vi "ifr2025 RF State.vi"(8 "error in (no error)":errorcluster {"code" format="%.0x"}, 9 "RF State (On)":bool=TRUE, 11 "instrument handle":refnum<visa-resource-name>) -> (0 "error out":errorcluster {"code" format="%.0x"}, 3 "instrument handle out":refnum<visa-resource-name>)   [LabVIEW 2009]
doc: "Controls the instrument RF output."
uses:
  Ifr2025_32.dll
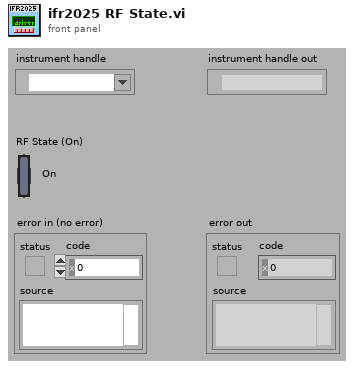
[diagram p1: front panel]
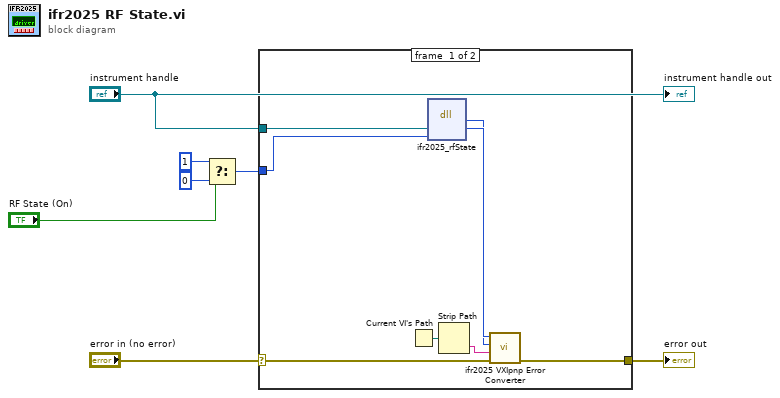
[diagram p0: block diagram]
diagram:
  n1 = Select(t=i16 1, s="RF State (On)", f=i16 0) -> (s? t:f=w1:i16)
  n2 = case shown="No Error" "error in (no error)" {
    selector: "error in (no error)" -> [w10 w16]
    tunnel: [w9 w16] -> w7
    tunnel: "instrument handle" -> [w14 _]
    tunnel: w1 -> [w8 _]
    frame #0 {
      n3 = Current VI's Path() -> (path=w15:path)
      n4 = dll-call lib="P:/inst/Marconi 2024 Signal Generator/source/labview/ifr2025/ifr2025/ifr2025_*.*" fn="ifr2025_rfState"("vi"=w14, "RF State"=w8) -> (w12:i32, "vi"=w13:u32)  [unwired: 4 in, 2 out]
      n5 = Strip Path(path=w15) -> (name=w11:string)  [unwired: 1 out]
      n6 = call "ifr2025 VXIpnp Error Converter.vi"("error in (no error)"=w10, "name of VI (\"\")"=w11, "CVI error code (0)"=w12, "instrument handle"=w13) -> ("error out"=w9:errorcluster)  [unwired: 7 out]
    }
    frame #1 {
    }
  }
  "error out" <- w7
  "instrument handle out" <- "instrument handle"
